vi "Assign GUID.vi"(8 "error in (no error)":errorcluster, 10 "GUID (optional)":string, 11 "Messenger in":refnum<class "Messenger.lvclass">) -> (0 "error out":errorcluster, 3 "Messenger out":refnum<class "Messenger.lvclass">)   [LabVIEW 2014, in "Messenger.lvclass"]
uses:
  Messenger.lvclass
  <vilib>/GPower/VIRegister/Library/Typedefs/RegisterType.ctl
  Messenger.lvclass/Messenger.ctl
  <vilib>/GPower/String/Library/RandomString.vi
  <vilib>/GPower/VIRegister/Library/QManager/CreateRegister.vi
  <vilib>/GPower/VIRegister/Library/QManager/QManagerAction.vi
  <vilib>/GPower/VIRegister/Library/QManager/GetQName.vi
  <vilib>/GPower/VIRegister/Library/QManager/StartQManager.vi
  <vilib>/GPower/VIRegister/VIRegister.lvlib
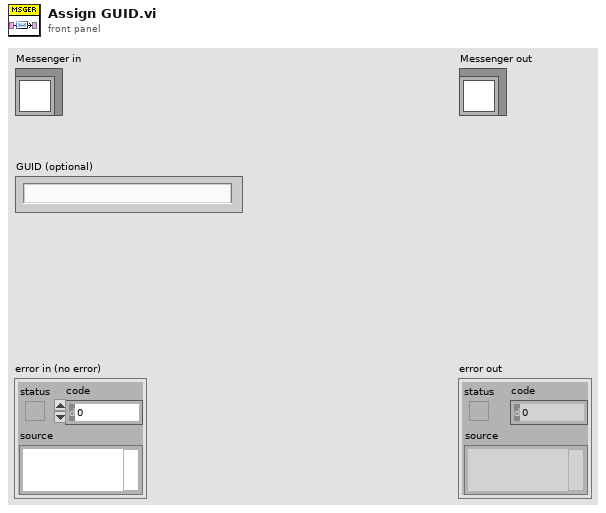
[diagram p1: front panel]
types:
  T1 = typedef "VIRegister.lvlib/RegisterType.ctl" = enum16{"Circular buffer", "FIFO buffer", "LIFO buffer", "Register"}
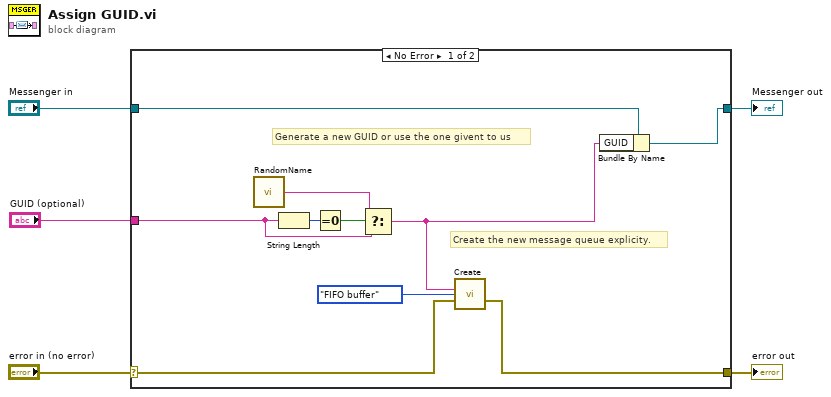
[diagram p0: block diagram]
diagram:
  n1 = case shown="No Error" "error in (no error)" {
    selector: "error in (no error)" -> [w7 w17]
    tunnel: [w6 w17] -> w4
    tunnel: [w14 w16] -> w2
    tunnel: "Messenger in" -> [w15 w16]
    tunnel: "GUID (optional)" -> [w11 _]
    frame No Error {
      # "Generate a new GUID or use the one givent to us"
      # "Create the new message queue explicity."
      n2 = call <vilib>:"RandomName.vi"() -> ("Random register name"=w10:string)
      n3 = String Length(string=w11) -> (length=w13:i32)
      n4 = Equal To 0?(x=w13) -> (x = 0?=w12:bool)
      n5 = Select(t=w10, s=w12, f=w11) -> (s? t:f=w9:string)
      n6 = call <vilib>:"Create.vi"("Register name"=w9, "Register type"=RegisterType."FIFO buffer", "Error in"=w7) -> ("Error out"=w6:errorcluster)  [unwired: 11 in, 1 out]
      n7 = Bundle By Name(cluster=w15, "GUID"=w9) -> (w14:refnum<class "Messenger.lvclass">)
    }
    frame Error {
    }
  }
  "error out" <- w4
  "Messenger out" <- w2
